vi "Enable-Disable Control-Indicator.vi"(7 "Control/Indicator Reference":refnum<vi>, 8 "error in (no error)":errorcluster, 11 "Enable/Disable":T1(ring)) -> (0 "error out":errorcluster)   [LabVIEW 2020]
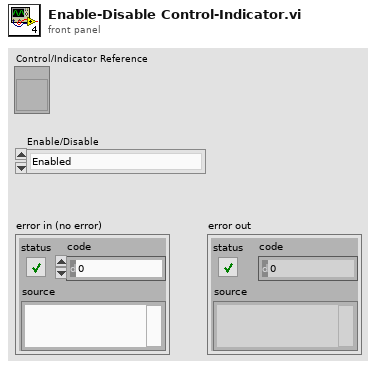
[diagram p1: front panel]
types:
  T1 = enum8{"Enabled", "Disabled", "Disabled and Grayed Out"}
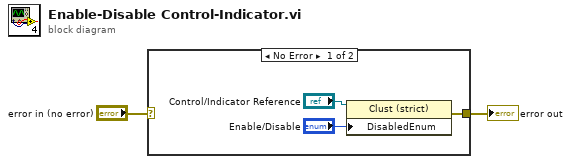
[diagram p0: block diagram]
diagram:
  n1 = case shown="No Error" "error in (no error)" {
    selector: "error in (no error)" -> [_ w6]
    tunnel: [w5 w6] -> w2
    frame No Error {
      n2 = property class="Clust (strict)"(reference="Control/Indicator Reference", "DisabledEnum"="Enable/Disable") -> (error out=w5:errorcluster)  [unwired: 1 in, 1 out]
    }
    frame Error {
    }
  }
  "error out" <- w2
